vi "Execute InPlaceElemNode Handle.vi"(4 "Menu Item Tag Suffix":string, 8 "错误输入（无错误）":errorcluster, 11 "元素同址操作节点输入":refnum<vi>) -> (0 "错误输出":errorcluster)   [LabVIEW 2020]
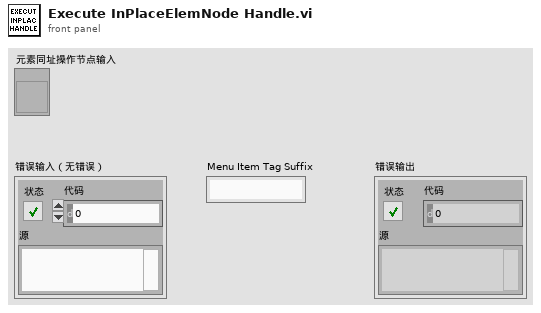
[diagram p1: front panel]
types:
  T1 = typedef "LVRectTypeDef.ctl" = cluster{"Left":i16, "Top":i16, "Right":i16, "Bottom":i16}
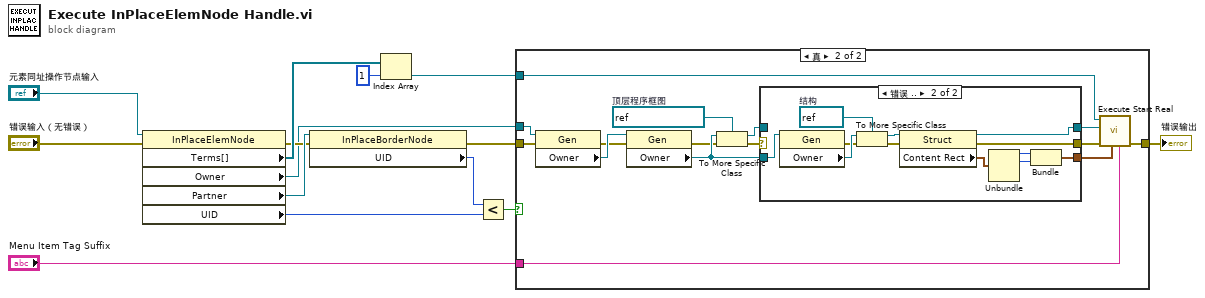
[diagram p0: block diagram]
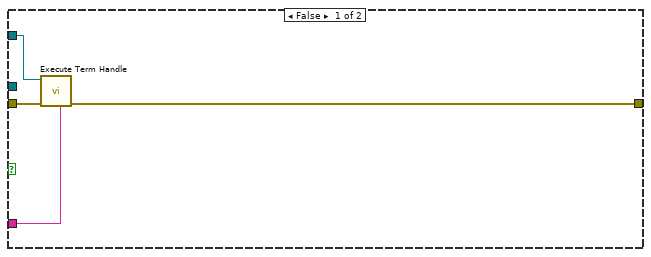
[diagram p2: hidden frame]
diagram:
  n1 = property class="InPlaceElemNode"(reference="元素同址操作节点输入", error in="错误输入（无错误）") -> (error out=w5:errorcluster, "Terms[]"=w10:refnum<vi>[], "Owner"=w1:refnum<vi>, "Partner"=w8:refnum<vi>, "UID"=w3:i32)  [unwired: 1 out]
  n2 = property class="InPlaceBorderNode"(reference=w8, error in=w5) -> (error out=w2:errorcluster, "UID"=w4:i32)  [unwired: 1 out]
  n3 = Index Array(array=w10, index=1 ("索引")) -> (element=w12:refnum<vi>)
  n4 = Less?(x=w4, y=w3) -> (x < y?=w9:bool)
  n5 = case shown="真" w9 {
    tunnel: w12 -> [w18 w20]
    tunnel: "Menu Item Tag Suffix" -> [w17 w19]
    tunnel: w1 -> [_ w33]
    tunnel: [w16 w21] -> w14
    tunnel: w2 -> [w15 w24]
    frame False {
      n6 = call "Execute Term Handle.vi"("Menu Item Tag Suffix"=w17, "错误输入（无错误）"=w15, "接线端输入"=w18) -> ("错误输出"=w16:errorcluster)  [unwired: 8 in]
    }
    frame True {
      w31 = refnum<vi> refnum  # 顶层程序框图
      n7 = property class="Gen"(reference=w33, error in=w24) -> (error out=w23:errorcluster, "Owner"=w32:refnum<vi>)  [unwired: 1 out]
      n8 = property class="Gen"(reference=w32, error in=w23) -> (error out=w22:errorcluster, "Owner"=w25:refnum<vi>)  [unwired: 1 out]
      n9 = To More Specific Class(target class=w31, reference=w25, error in=w22) -> (specific class reference=w28:refnum<vi>, error out=w30:errorcluster)
      n10 = case shown="错误 .." w30 {
        selector: w30 -> [w34 _]
        tunnel: w25 -> [_ w47]
        tunnel: [_ w39] -> w27
        tunnel: [w35 w40] -> w29
        tunnel: w28 -> [w35 _]
        tunnel: [w34 w36] -> w26
        frame No Error {
        }
        frame Error {
          w46 = refnum<vi> refnum  # 结构
          n11 = property class="Gen"(reference=w47) -> (error out=w38:errorcluster, "Owner"=w45:refnum<vi>)  [unwired: 1 in, 1 out]
          n12 = To More Specific Class(target class=w46, reference=w45, error in=w38) -> (specific class reference=w44:refnum<vi>, error out=w37:errorcluster)
          n13 = property class="Struct"(reference=w44, error in=w37) -> (reference out=w40:refnum<vi>, error out=w36:errorcluster, "Content Rect"=w41:T1)
          n14 = Unbundle(w41) -> ("Left"=w43:i16, "Top"=w42:i16)  [unwired: 2 out]
          n15 = Bundle("Left"=w43, "Top"=w42) -> (w39:cluster{"Left":i16, "Top":i16})  [unwired: 1 in]
        }
      }
      n16 = call "Execute Start Real.vi"("Menu Item Tag Suffix"=w19, "相对位置原点"=w27, "错误输入（无错误）"=w26, "所有者引用句柄"=w29, "接线端输入"=w20) -> ("错误输出"=w21:errorcluster)  [unwired: 6 in]
    }
  }
  "错误输出" <- w14
